vi "QueryTemperature.vi"(6 "error":errorcluster, 9 "VISA resource name":refnum<visa-resource-name>) -> (0 "error out":errorcluster, 2 "Temperature (C)":i32, 3 "VISA resource name out":refnum<visa-resource-name>, 5 "Response":string)   [LabVIEW 2015, in "BigSkyControl.lvlib"]
uses:
  BigSkyControl.lvlib
panel:
  out "Read return count":u32
  in  "byte count":u32=1024
  out "Write return count":u32
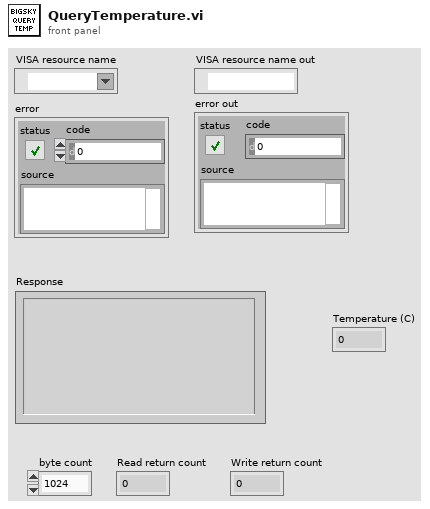
[diagram p1: front panel]
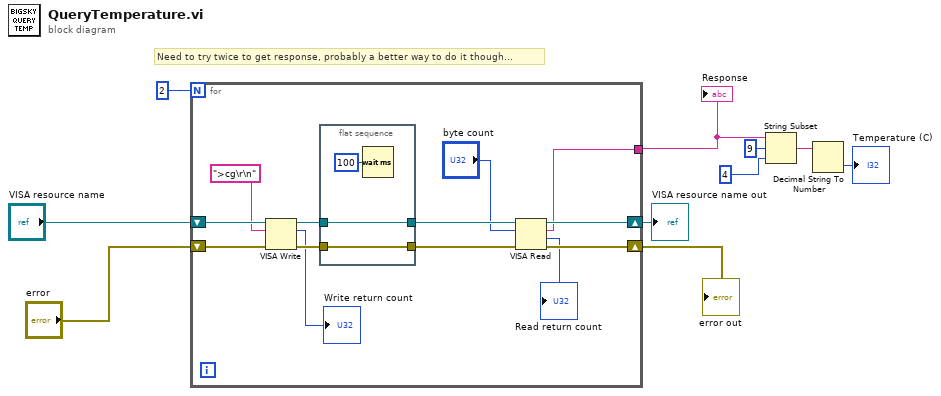
[diagram p0: block diagram]
diagram:
  # "Need to try twice to get response, probably a better way to do it though..."
  n1 = for {
    N: 2 -> [_]
    shift-right: [w22] -> w7
    shift-left: "VISA resource name" -> [w21]
    shift-right: [w23] -> w6
    shift-left: "error" -> [w20]
    tunnel: [w12] -> w5
    n2 = VISA Write(VISA resource name=w21, write buffer=">cg\r\n", error in (no error)=w20) -> (VISA resource name out=w18:refnum<visa-resource-name>, return count=→"Write return count":u32, error out=w19:errorcluster)
    n3 = flat-sequence {
      tunnel: w19 -> [w26]
      tunnel: [w26] -> w16
      tunnel: w18 -> [w25]
      tunnel: [w25] -> w17
      frame #0 {
        n4 = Wait (ms)(milliseconds to wait=u32 100) -> ()  [unwired: 1 out]
      }
    }
    n5 = VISA Read(VISA resource name=w17, byte count="byte count", error in (no error)=w16) -> (VISA resource name out=w22:refnum<visa-resource-name>, read buffer=w12:string, return count=→"Read return count":u32, error out=w23:errorcluster)
  }
  "Response" <- w5
  "VISA resource name out" <- w7
  "error out" <- w6
  n6 = String Subset(string=w5, offset (0)=9, length (rest)=4 ("length (rest)")) -> (substring=w2:string)
  n7 = Decimal String To Number(string=w2) -> (number=→"Temperature (C)":i32)  [unwired: 2 in, 1 out]
